vi "Append Circumnavigate Waypoint.vi"(0 "Waypoint Array In":T1[](array[typedef]), 5 "Lat":sgl, 7 "Lon":sgl, 9 "Altitude (m)":sgl, 11 "Error In":errorcluster, 12 "Circumnavigate radius (m)":sgl, 13 "Capture Photo":bool) -> (4 "appended array":T1[](array[typedef]), 15 "Error Out":errorcluster)   [LabVIEW 2014]
uses:
  Controls/Mission Planning Controls/MAVLINK Mission Item.ctl
  Controls/MAVLINK Mav Frame.ctl
  Commands/Mission Planning/MISSION_ITEM SubVI/MISSION_ITEM Set ROI.vi
  Commands/Mission Planning/MISSION_ITEM SubVI/MISSION_ITEM Loiter (Turns).vi
  Commands/Mission Planning/MISSION_ITEM SubVI/MISSION_ITEM Set Circle Radius.vi
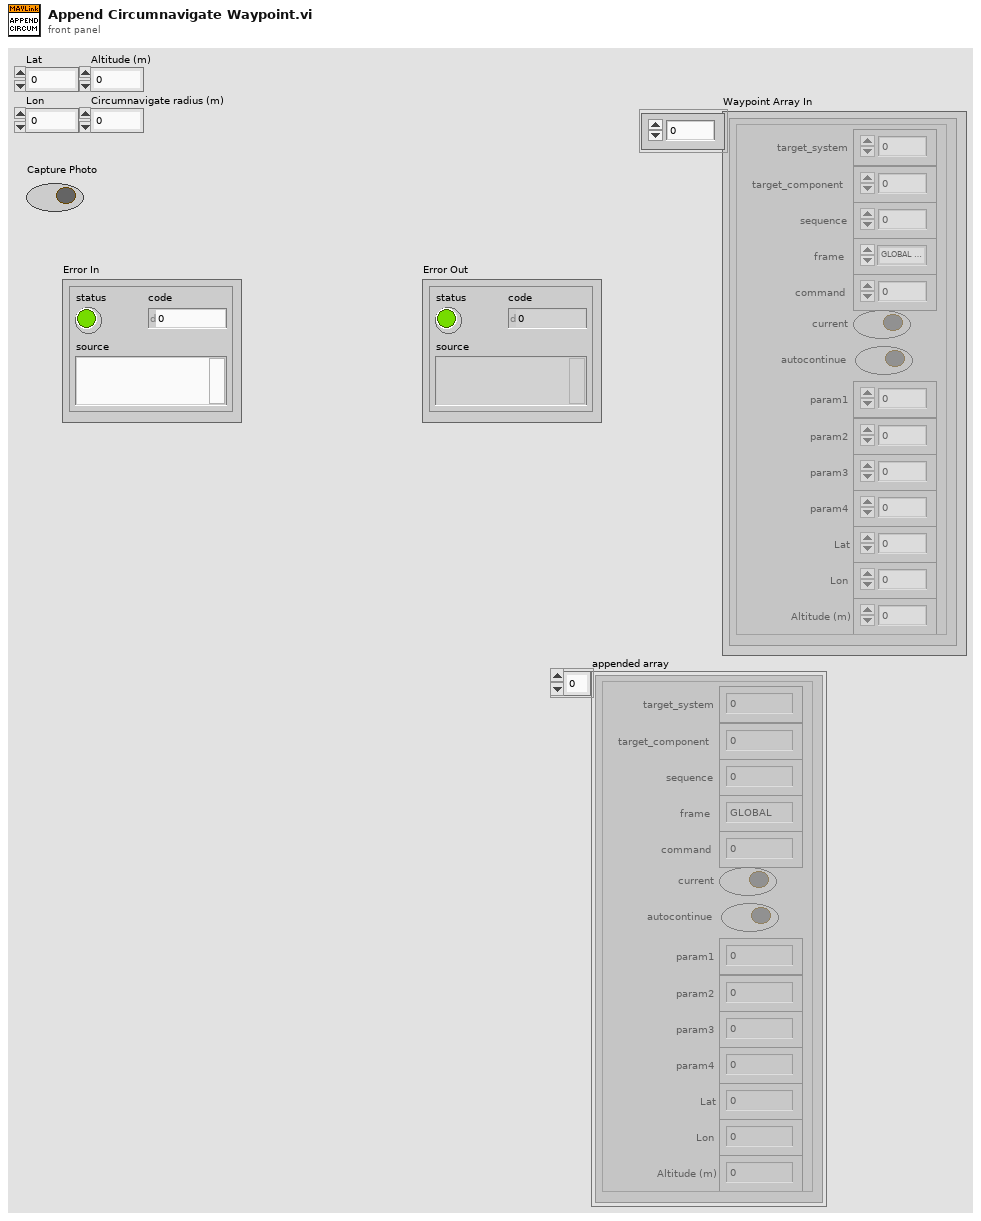
[diagram p1: front panel]
types:
  T1 = typedef "MAVLINK Mission Item.ctl" = cluster{"target_system":u8, "target_component":u8, "sequence":u16, "frame":T2, "command":u16, "current":bool, "autocontinue":bool, "param1":sgl, "param2":sgl, "param3":sgl, "param4":sgl, "Lat":sgl, "Lon":sgl, "Altitude (m)":sgl}
  T2 = typedef "MAVLINK Mav Frame.ctl" = enum8{"GLOBAL", "LOCAL NED", "MISSION", "GLOBAL RELATIVE ALT", "LOCAL ENU", "GLOBAL INT", "GLOBAL RELATIVE ALT INT", "LOCAL OFFSET NED", "BODY NED", "BODY OFFSET NED", "GLOBAL TERRAIN ALT", "GLOBAL TERRAIN ALT INT"}
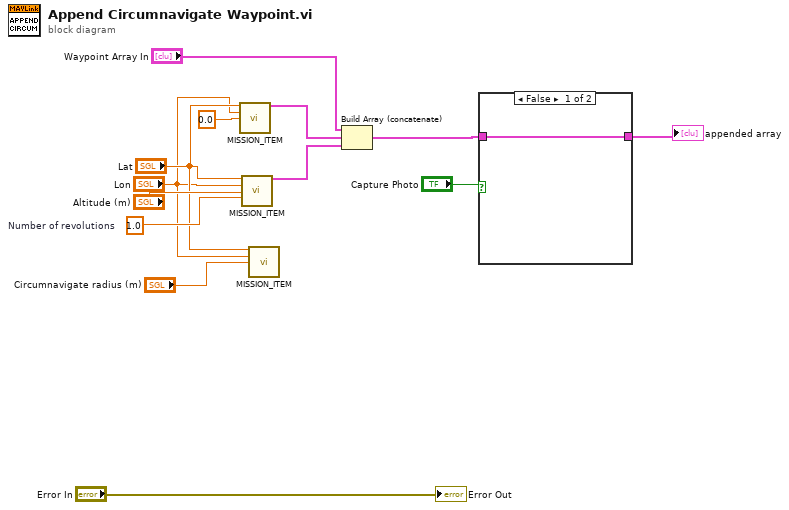
[diagram p0: block diagram]
diagram:
  w7 = sgl 1.0  # Number of revolutions
  n1 = call-poly "MISSION_ITEM.vi"("Lat"="Lat", "Lon"="Lon", "Altitude (m)"=sgl 0.0 ("Lat")) -> ("Mission Item"=w9:T1)  [unwired: 12 in]
  n2 = call-poly "MISSION_ITEM.vi"("Lat"="Lat", "Lon"="Lon", "Altitude (m)"="Altitude (m)", "Number of revolutions"=w7) -> ("Mission Item"=w11:T1)  [unwired: 11 in]
  n3 = call-poly "MISSION_ITEM.vi"("Lat"="Lat", "Lon"="Lon", "Circle Radius (m)"="Circumnavigate radius (m)") -> ()  [unwired: 12 in, 1 out]
  n4 = Build Array (concatenate)("Waypoint Array In", w9, w11) -> (w3:T1[])
  n5 = case shown="False" "Capture Photo" {
    tunnel: w3 -> [w14 w15]
    tunnel: [w14 w15] -> w1
    frame False {
    }
    frame True {
    }
  }
  "appended array" <- w1
  "Error Out" <- "Error In"
